vi "PCO_GetCameraDescription2.vi"(8 "error in (no error)":errorcluster {"code" format="%x"}, 11 "ph":u64) -> (0 "error out":errorcluster {"code" format="%x"}, 1 "strDescription":T1 {"dwModulateCapsDESC2" format="%x"}, 2 "ErrorMessage":i32 format="%x", 3 "ph out":u64)   [LabVIEW 2019, in "SDK.lvlib" / "CameraDescription.lvlib"]
doc: "<b>Description:</b>\nAny of the available sensor and camera specific description can be queried. With input parameter wType the returned description structure can be selected. PCO_DescriptionEx is a generic structure which has to be casted to/from the queried structure. The wSize parameter has to be filled with the correct value for the requested structure. This function was introduced due to the size limitation of the standard camera descriptor and the need for describing additional features.\n\n<b>Supported camera type:</b>\nAll cameras\n\n<b>Descriptor dependency:</b>\ndwGeneralCapsDESC1: ENHANCED_DESCRIPTOR_2"
uses:
  CameraDescription.lvlib
  Structures/Structures.lvlib
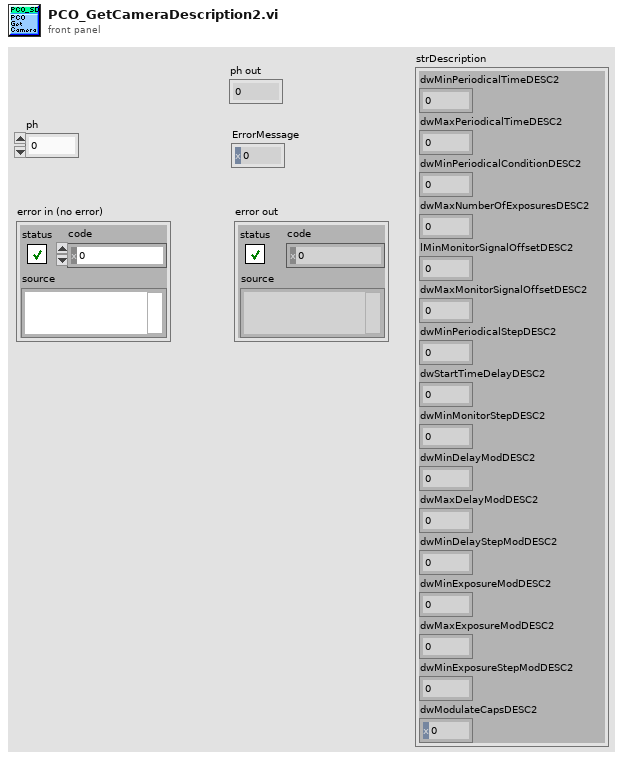
[diagram p1: front panel]
types:
  T1 = cluster{"dwMinPeriodicalTimeDESC2":u32, "dwMaxPeriodicalTimeDESC2":u32, "dwMinPeriodicalConditionDESC2":u32, "dwMaxNumberOfExposuresDESC2":u32, "lMinMonitorSignalOffsetDESC2":i32, "dwMaxMonitorSignalOffsetDESC2":u32, "dwMinPeriodicalStepDESC2":u32, "dwStartTimeDelayDESC2":u32, "dwMinMonitorStepDESC2":u32, "dwMinDelayModDESC2":u32, "dwMaxDelayModDESC2":u32, "dwMinDelayStepModDESC2":u32, "dwMinExposureModDESC2":u32, "dwMaxExposureModDESC2":u32, "dwMinExposureStepModDESC2":u32, "dwModulateCapsDESC2":u32}
  T2 = cluster{"wSize":u16, "ZZwAlignDummy1":u16, "dwMinPeriodicalTimeDESC2":u32, "dwMaxPeriodicalTimeDESC2":u32, "dwMinPeriodicalConditionDESC2":u32, "dwMaxNumberOfExposuresDESC2":u32, "lMinMonitorSignalOffsetDESC2":i32, "dwMaxMonitorSignalOffsetDESC2":u32, "dwMinPeriodicalStepDESC2":u32, "dwStartTimeDelayDESC2":u32, "dwMinMonitorStepDESC2":u32, "dwMinDelayModDESC2":u32, "dwMaxDelayModDESC2":u32, "dwMinDelayStepModDESC2":u32, "dwMinExposureModDESC2":u32, "dwMaxExposureModDESC2":u32, "dwMinExposureStepModDESC2":u32, "dwModulateCapsDESC2":u32, "dwReserved":cluster{u32, u32, u32, u32, u32, u32, u32, u32, u32, u32, u32, u32, u32, u32, u32, u32}, "ZZdwDummy":cluster{u32, u32, u32, u32, u32, u32, u32, u32, u32, u32, u32, u32, u32, u32, u32, u32, u32, u32, u32, u32, u32, u32, u32, u32, u32, u32, u32, u32, u32, u32, u32, u32, u32, u32, u32, u32, u32, u32, u32, u32, u32}}
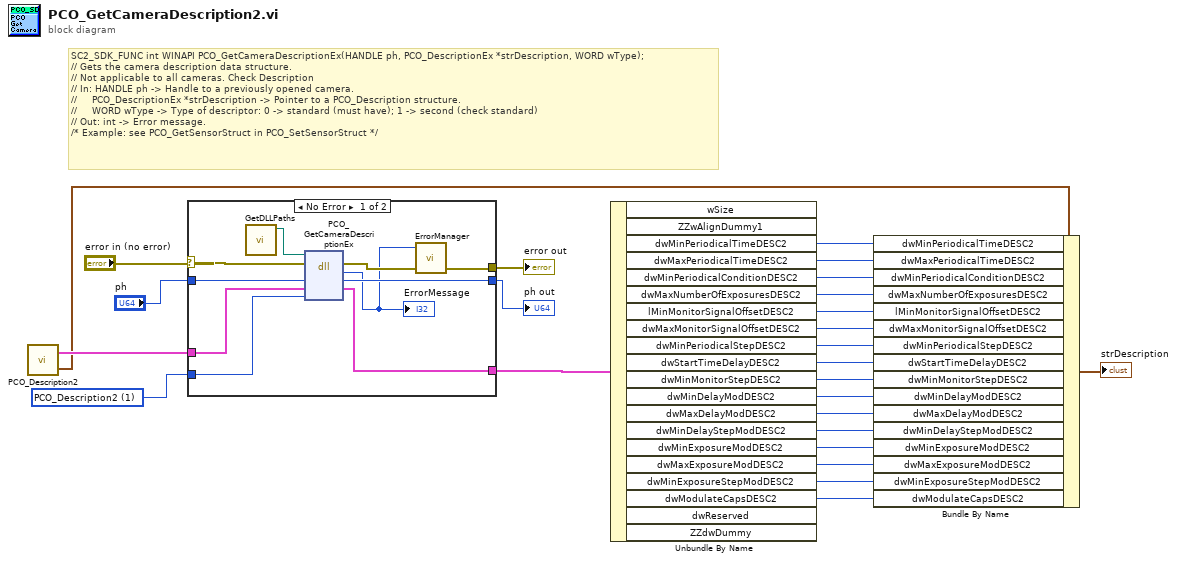
[diagram p0: block diagram]
diagram:
  w1 = u16 1 items=["PCO_Description", "PCO_Description2"] ("wType")
  # "SC2_SDK_FUNC int WINAPI PCO_GetCameraDescriptionEx(HANDLE ph, PCO_DescriptionEx *strDescription, WORD wType);\n// Gets the camera description data structure.\n// Not applicable to all cameras. Check Description\n// In: HANDLE ph -> Handle to a previously opened camera.\n//     PCO_DescriptionEx *strDescription -> Pointer to a PCO_Description structure.\n//     WORD wType -> Type of descriptor: 0 -> standard (must have); 1 -> second (check standard)\n// Out: int -> Error message.\n/* Example: see PCO_GetSensorStruct in PCO_SetSensorStruct */"
  n1 = call "PCO_Description2.vi"() -> ("PCO_Description2"=w19:T1, "PCO_Description2_Raw"=w21:T2)  [unwired: 4 in, 2 out]
  n2 = case shown="No Error" "error in (no error)" {
    selector: "error in (no error)" -> [w34 w38]
    tunnel: "ph" -> [w35 w37]
    tunnel: w21 -> [w29 w36]
    tunnel: [w31 w38] -> w23
    tunnel: [w33 w37] -> w22
    tunnel: [w28 w36] -> w20
    tunnel: w1 -> [w27 _]
    frame No Error {
      n3 = call "GetDLLPaths.vi"() -> ("SC2_Cam_Path"=w26:path)  [unwired: 9 in, 2 out]
      n4 = dll-call lib="?" fn="PCO_GetCameraDescriptionEx"(path in=w26, error in=w34, "ph"=w35, "strDescription"=w29, "wType"=w27) -> (error out=w32:errorcluster, "return type"=w30:i32, "ph"=w33:u64, "strDescription"=w28:T2)  [unwired: 2 in, 1 out]
      "ErrorMessage" <- w30
      n5 = call "ErrorManager.vi"("error in (no error)"=w32, "error code"=w30) -> ("error out"=w31:errorcluster)  [unwired: 3 in]
    }
    frame Error {
    }
  }
  "error out" <- w23
  "ph out" <- w22
  n6 = Unbundle By Name(w20) -> ("dwMinPeriodicalTimeDESC2"=w18:u32, "dwMaxPeriodicalTimeDESC2"=w17:u32, "dwMinPeriodicalConditionDESC2"=w16:u32, "dwMaxNumberOfExposuresDESC2"=w15:u32, "lMinMonitorSignalOffsetDESC2"=w14:i32, "dwMaxMonitorSignalOffsetDESC2"=w13:u32, "dwMinPeriodicalStepDESC2"=w12:u32, "dwStartTimeDelayDESC2"=w11:u32, "dwMinMonitorStepDESC2"=w10:u32, "dwMinDelayModDESC2"=w9:u32, "dwMaxDelayModDESC2"=w8:u32, "dwMinDelayStepModDESC2"=w7:u32, "dwMinExposureModDESC2"=w6:u32, "dwMaxExposureModDESC2"=w5:u32, "dwMinExposureStepModDESC2"=w4:u32, "dwModulateCapsDESC2"=w3:u32)  [unwired: 4 out]
  n7 = Bundle By Name(cluster=w19, "dwMinPeriodicalTimeDESC2"=w18, "dwMaxPeriodicalTimeDESC2"=w17, "dwMinPeriodicalConditionDESC2"=w16, "dwMaxNumberOfExposuresDESC2"=w15, "lMinMonitorSignalOffsetDESC2"=w14, "dwMaxMonitorSignalOffsetDESC2"=w13, "dwMinPeriodicalStepDESC2"=w12, "dwStartTimeDelayDESC2"=w11, "dwMinMonitorStepDESC2"=w10, "dwMinDelayModDESC2"=w9, "dwMaxDelayModDESC2"=w8, "dwMinDelayStepModDESC2"=w7, "dwMinExposureModDESC2"=w6, "dwMaxExposureModDESC2"=w5, "dwMinExposureStepModDESC2"=w4, "dwModulateCapsDESC2"=w3) -> (→"strDescription":T1)
